vi "系统设置.vi"() -> ()   [LabVIEW 2016]
uses:
  <vilib>/Utility/miscctls.llb/LVPointTypeDef.ctl
  <vilib>/ptbypt/NI_PtbyPt.lvlib
  <vilib>/Utility/config.llb/NI_LVConfig.lvlib
  PLC/PLC.lvlib
panel:
  in  "CODCr":bool
  in  "总磷总氮":bool
  in  "氨氮":bool
  in  "CODmn":bool
  in  "多参数":bool
  in  "24H周期设置":bool[](xcontrol)
  in  "输入密码":dbl
  in  "布尔":bool
  in  "副屏设置":bool
  in  "开机启动":bool caption="氨氮禁用"
  in  "CODMn启用":bool caption="CODMn禁用"
  in  "质控单元启用":bool caption="质控单元禁用"
  in  "总磷总氮启用":bool caption="总磷总氮禁用"
  in  "流量计启用":bool caption="流量计禁用"
  in  "氨氮启用":bool caption="氨氮禁用"
  in  "多参数启用":bool caption="多参数禁用"
  in  "CODcr启用":bool caption="CODcr禁用"
  in  "运行模式":enum16{"维护模式", "常规模式", "应急模式", "质控模式"}(ring)
  # "自动运行启动参数"
  # "启动周期设置"
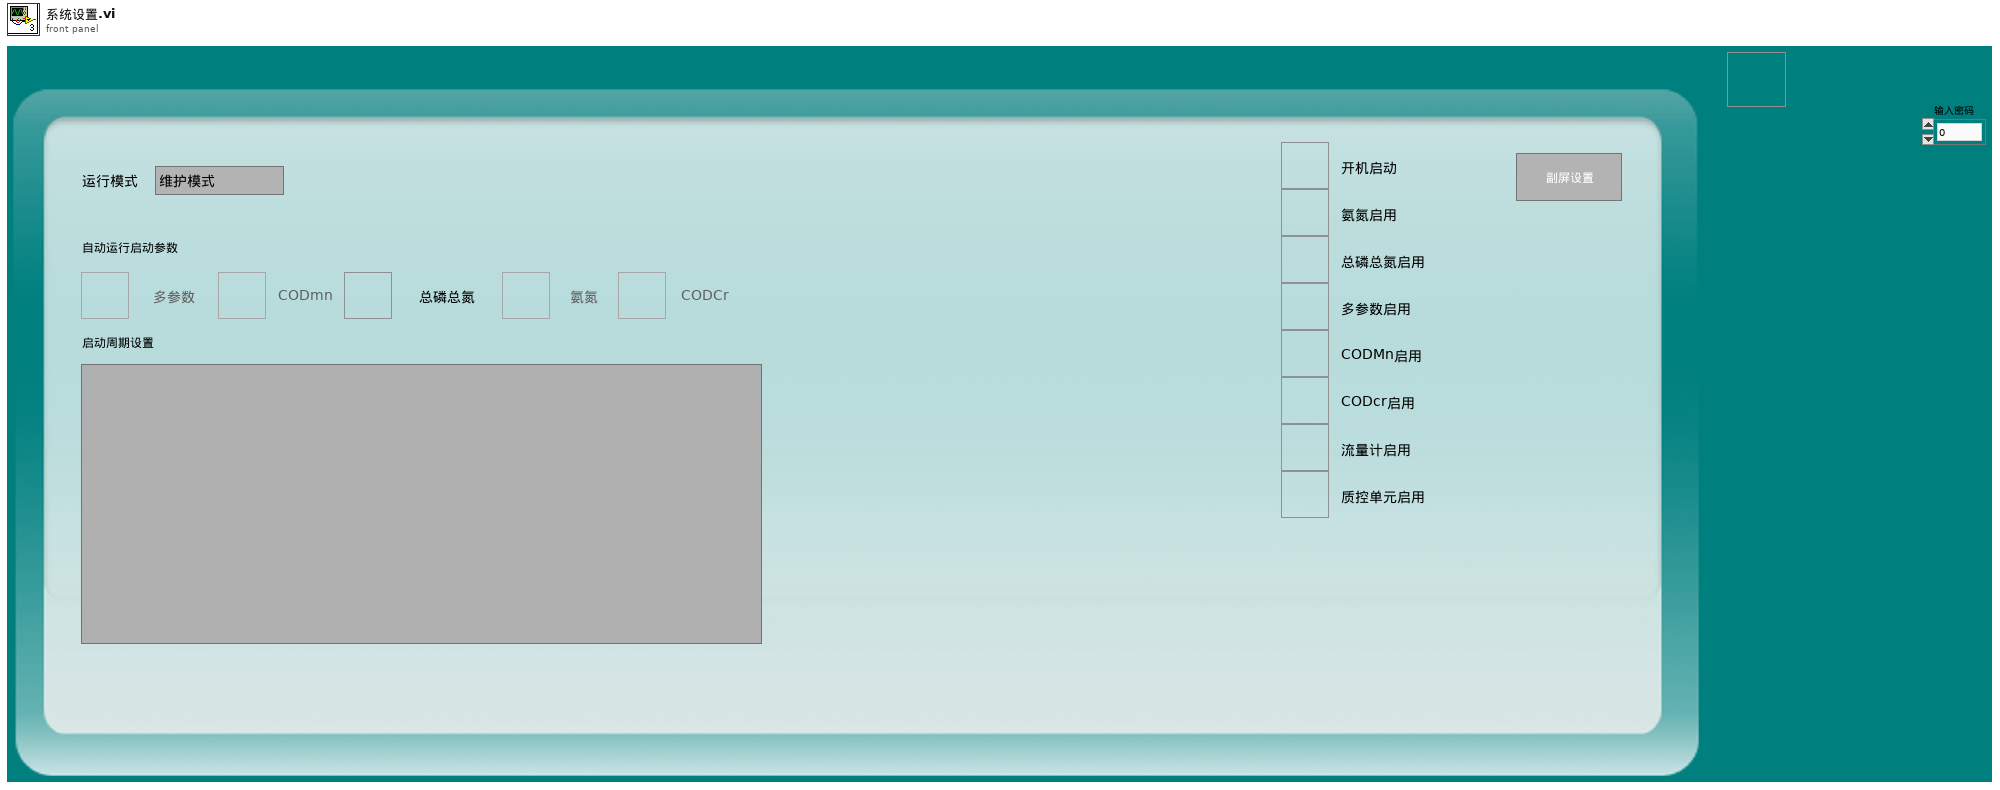
[diagram p1: front panel]
types:
  T1 = typedef "LVPointTypeDef.ctl" = cluster{"Horizontal":i16, "Vertical":i16}
  T2 = typedef "NI_LVConfig.lvlib/Config Data RefNum.ctl" = refnum<k1>
  T3 = enum8{"Enabled", "Disabled", "Disabled and Grayed Out"}
  T4 = cluster{"运行模式":enum16{"维护模式", "常规模式", "应急模式", "质控模式"}}
  T5 = cluster{"测量模式":enum16{"水样测量", "标样核查", "零点核查", "加标回收", "平行样", "校零", "校标"}}
  T6 = cluster{"CODCr":cluster{"启动测量模式":cluster{"测量模式":enum16{"水样测量", "标样核查", "零点核查", "加标回收", "平行样", "校零", "校标"}}, "确定按钮":bool}, "参数启用":cluster{"多参数":bool, "CODMn":bool, "总磷总氮":bool, "氨氮":bool, "CODcr":bool}}
  T7 = typedef "LVDateTimeRec.ctl" = cluster{"秒数的小数部分":dbl, "秒":i32, "分":i32, "时":i32, "日":i32, "月":i32, "年":i32, "天数（周）":i32, "天数（年）":i32, "DST":i32}
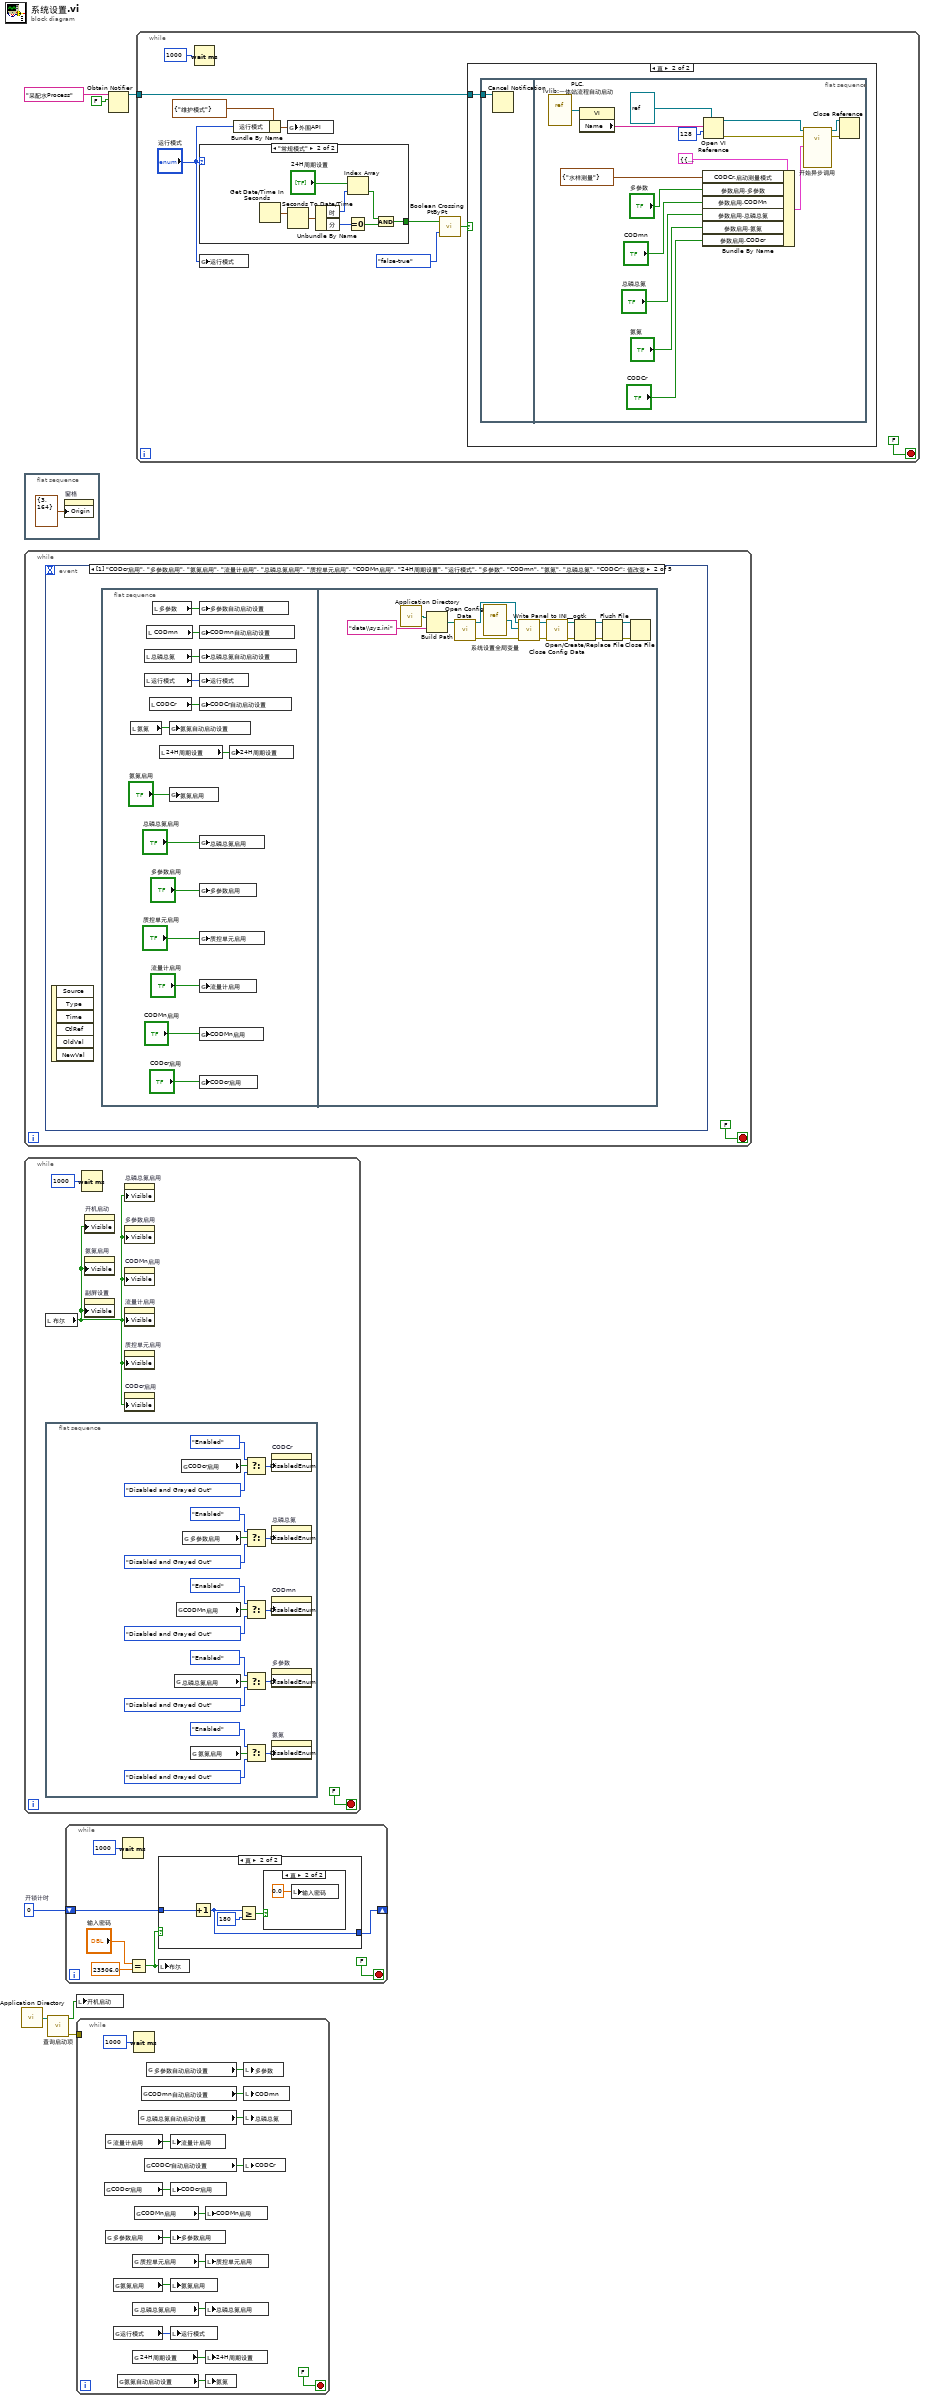
[diagram p0: block diagram]
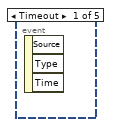
[diagram p6: hidden frame]
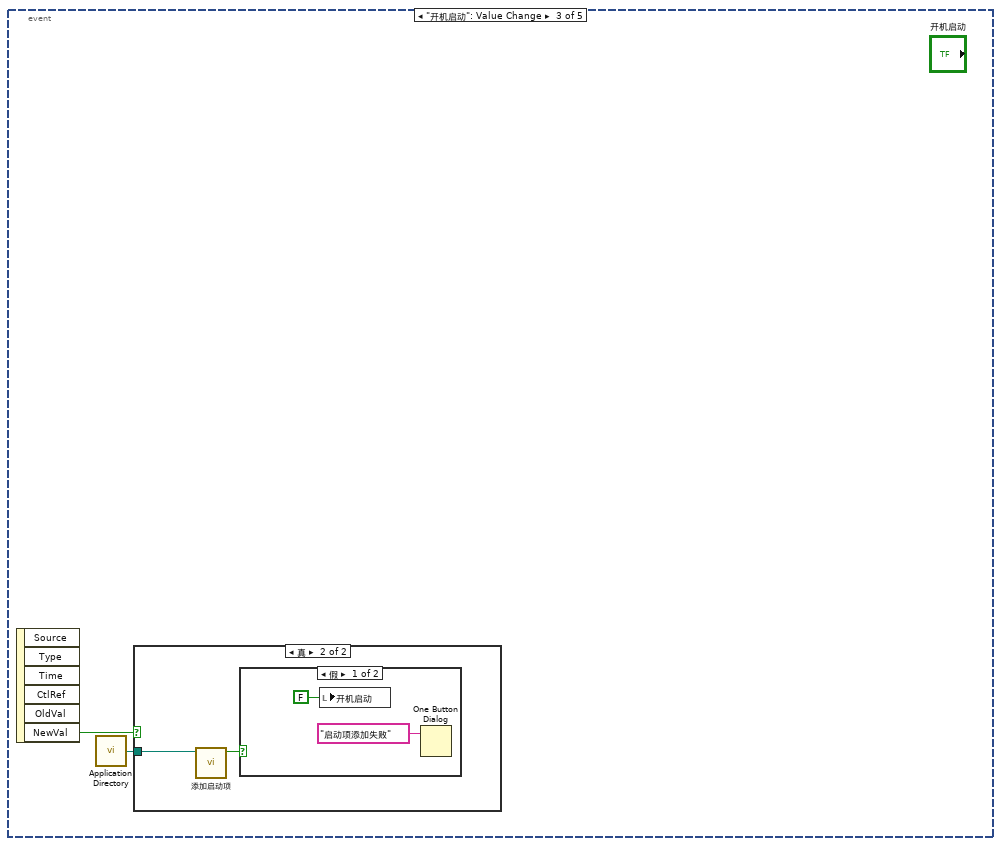
[diagram p7: hidden frame]
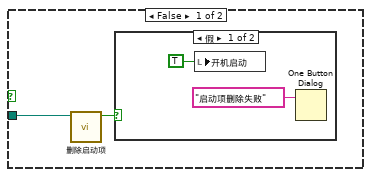
[diagram p8: hidden frame]
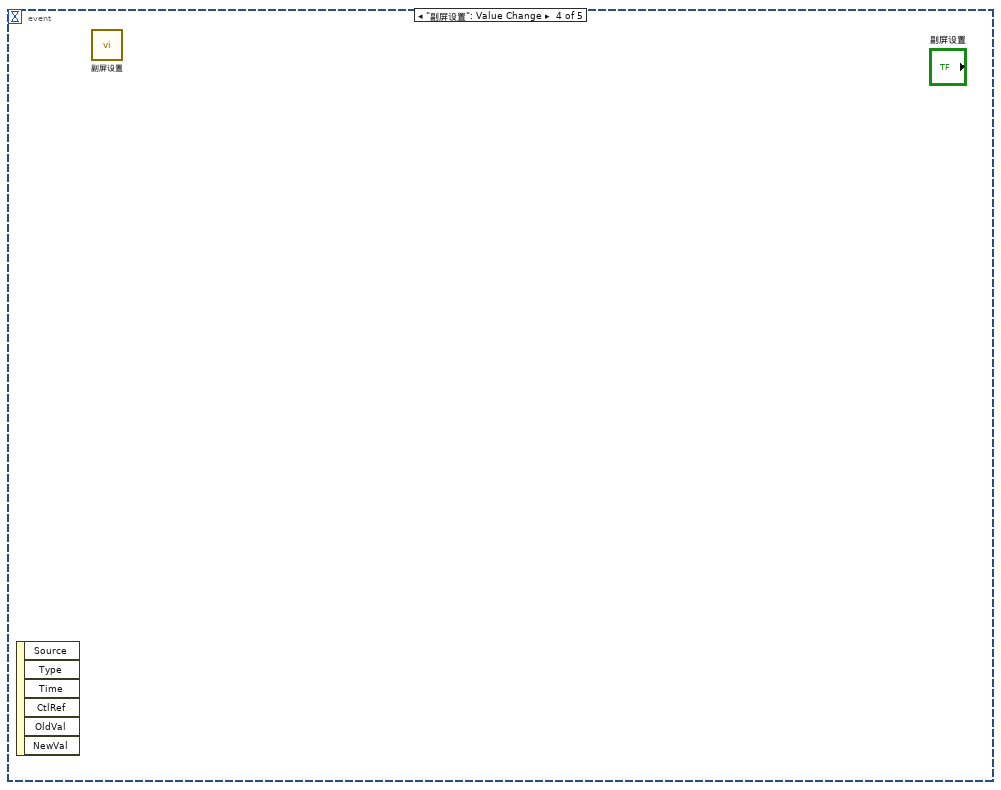
[diagram p11: hidden frame]
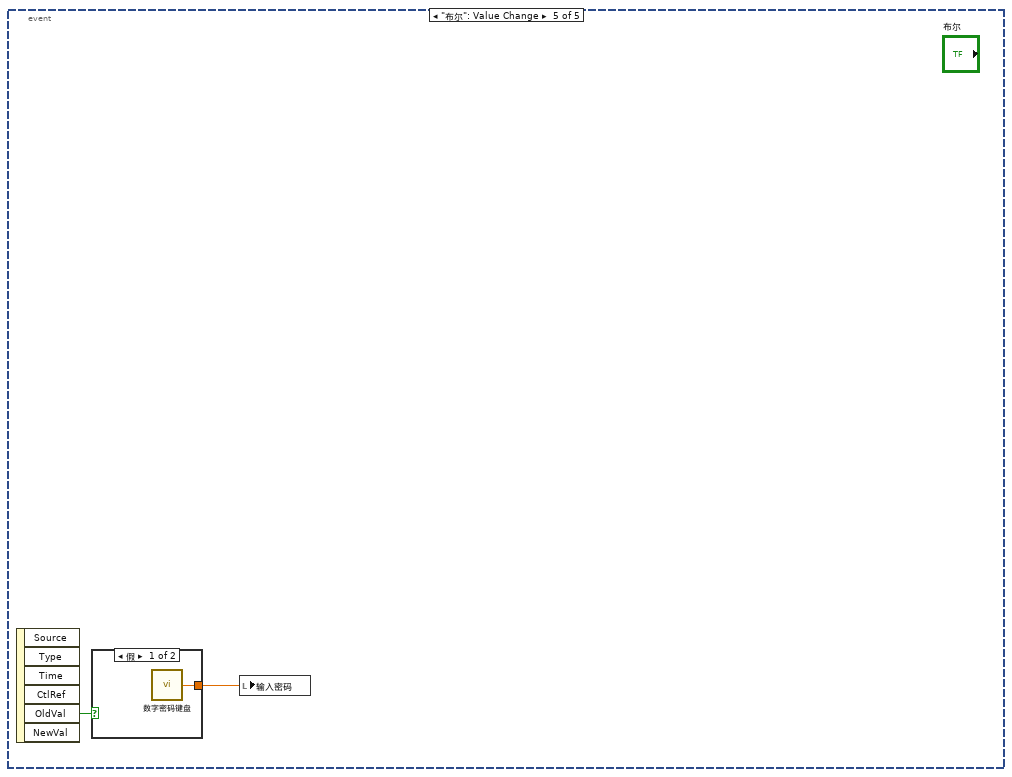
[diagram p12: hidden frame]
diagram:
  w1 = u32 0  # 开锁计时
  n1 = call <vilib>:"Application Directory.vi"() -> ("Application Directory"=w4:path)
  n2 = flat-sequence {
    frame #0 {
      n3 = property on="窗格" class="Pane"("Origin"=T1 {"Horizontal"=3, "Vertical"=164} ("原点")) -> ()  [unwired: 2 in, 2 out]
    }
  }
  n4 = while {
    stop <- FALSE stop-if-true
    n5 = event shown="[1] \"CODcr启用\", \"多参数启用\", \"氨氮启用\", \"流量计启用\", \"总磷总氮启用\", \"质控单元启用\", \"CODMn启用\", \"24H周期设置\", \"运行模式\", \"多参数\", \"CODmn\", \"氨氮\", \"总磷总氮\", \"CODCr\": 值改变" {
      selector: _ -> [_ _ _ _ _]
      dyn-events: _ -> [_ _ _ _ _]
      timeout: _ -> [_ _ _ _ _]
      event Timeout {
        n6 = event-data() -> ()  [unwired: 1 in, 3 out]
      }
      event "CODcr启用", "多参数启用", "氨氮启用", "流量计启用", "总磷总氮启用", "质控单元启用", "CODMn启用", "24H周期设置", "运行模式", "多参数", "CODmn", "氨氮", "总磷总氮", "CODCr": Value Change {
        n7 = event-data() -> ()  [unwired: 1 in, 6 out]
        n8 = flat-sequence {
          frame #0 {
            n9 = local read "氨氮"() -> (w14:bool)
            n10 = local read "总磷总氮"() -> (w12:bool)
            n11 = local read "运行模式"() -> (w15:enum16{"维护模式", "常规模式", "应急模式", "质控模式"})
            n12 = local read "CODmn"() -> (w11:bool)
            n13 = local read "CODCr"() -> (w13:bool)
            n14 = local read "多参数"() -> (w10:bool)
            n15 = local read "24H周期设置"() -> (w16:bool[])
            n16 = global write "系统设置全局变量.vi" "氨氮自动启动设置"(w14) -> ()
            n17 = global write "系统设置全局变量.vi" "氨氮启用"("氨氮启用") -> ()
            n18 = global write "系统设置全局变量.vi" "多参数自动启动设置"(w10) -> ()
            n19 = global write "系统设置全局变量.vi" "CODmn自动启动设置"(w11) -> ()
            n20 = global write "系统设置全局变量.vi" "总磷总氮自动启动设置"(w12) -> ()
            n21 = global write "系统设置全局变量.vi" "运行模式"(w15) -> ()
            n22 = global write "系统设置全局变量.vi" "CODCr自动启动设置"(w13) -> ()
            n23 = global write "系统设置全局变量.vi" "总磷总氮启用"("总磷总氮启用") -> ()
            n24 = global write "系统设置全局变量.vi" "多参数启用"("多参数启用") -> ()
            n25 = global write "系统设置全局变量.vi" "质控单元启用"("质控单元启用") -> ()
            n26 = global write "系统设置全局变量.vi" "流量计启用"("流量计启用") -> ()
            n27 = global write "系统设置全局变量.vi" "CODMn启用"("CODMn启用") -> ()
            n28 = global write "系统设置全局变量.vi" "CODcr启用"("CODcr启用") -> ()
            n29 = global write "系统设置全局变量.vi" "24H周期设置"(w16) -> ()
          }
          frame #1 {
            n30 = call <vilib>:"Application Directory.vi"() -> ("Application Directory"=w37:path)
            n31 = Build Path(base path=w37, name or relative path="data\\sys.ini" ("名称或相对路径")) -> (appended path=w35:path)
            n32 = call <vilib>:"Open Config Data.vi"("configuration file path"=w35) -> ("error out"=w31:errorcluster, "refnum"=w34:T2)  [unwired: 8 in, 1 out]
            n33 = vi-ref "系统设置全局变量.vi"() -> (w33:refnum<vi>)
            n34 = call <userlib>:"Write Panel to INI__ogtk.vi"("error in (no error)"=w31, "VI ref"=w33, "refnum"=w34) -> ("error out"=w30:errorcluster, "refnum out"=w32:T2)  [unwired: 7 in]
            n35 = call <vilib>:"Close Config Data.vi"("error in (no error)"=w30, "refnum"=w32) -> ("error out"=w25:errorcluster, "file path"=w24:path)  [unwired: 8 in]
            n36 = Open/Create/Replace File(file path (use dialog)=w24, error in=w25) -> (refnum out=w28:refnum<file>, error out=w29:errorcluster)  [unwired: 4 in, 1 out]
            n37 = Flush File(refnum=w28, error in=w29) -> (refnum out=w27:refnum<file>, error out=w26:errorcluster)
            n38 = Close File(refnum=w27, error in=w26) -> ()  [unwired: 2 out]
          }
        }
      }
      event "开机启动": Value Change {
        n39 = event-data() -> ("NewVal"=w39:bool)  [unwired: 1 in, 5 out]
        n40 = call <vilib>:"Application Directory.vi"() -> ("Application Directory"=w38:path)
        n41 = case shown="真" w39 {
          tunnel: w38 -> [w41 w45]
          frame False {
            n42 = call "删除启动项.vi"("启动文件路径"=w41) -> ("删除标记"=w40:bool)  [unwired: 9 in, 1 out]
            n43 = case shown="假" w40 {
              frame False {
                n44 = local write "开机启动"(TRUE ("开机启动")) -> ()
                n45 = One Button Dialog(message="启动项删除失败" ("消息")) -> ()  [unwired: 1 in, 1 out]
              }
              frame True {
              }
            }
          }
          frame True {
            n46 = call "添加启动项.vi"("启动文件路径"=w45) -> ("添加成功标记"=w44:bool)  [unwired: 9 in, 1 out]
            n47 = case shown="假" w44 {
              frame False {
                n48 = local write "开机启动"(FALSE ("开机启动")) -> ()
                n49 = One Button Dialog(message="启动项添加失败" ("消息")) -> ()  [unwired: 1 in, 1 out]
              }
              frame True {
              }
            }
          }
        }
      }
      event "副屏设置": Value Change {
        n50 = event-data() -> ()  [unwired: 1 in, 6 out]
        n51 = call "副屏设置.vi"() -> ()  [unwired: 12 in]
      }
      event "布尔": Value Change {
        n52 = event-data() -> ("OldVal"=w49:bool)  [unwired: 1 in, 5 out]
        n53 = case shown="假" w49 {
          tunnel: [w50 _] -> w48
          frame False {
            n54 = call "数字密码键盘.vi"() -> ("NewNumber"=w50:sgl)  [unwired: 1 in]
          }
          frame True {
          }
        }
        n55 = local write "输入密码"(w48) -> ()
      }
    }
  }
  n56 = while {
    stop <- FALSE stop-if-true
    n57 = local read "布尔"() -> (w51:bool)
    n58 = flat-sequence {
      frame #0 {
        n59 = global read "系统设置全局变量.vi" "总磷总氮启用"() -> (w58:bool)
        n60 = global read "系统设置全局变量.vi" "CODMn启用"() -> (w56:bool)
        n61 = global read "系统设置全局变量.vi" "CODcr启用"() -> (w57:bool)
        n62 = global read "系统设置全局变量.vi" "多参数启用"() -> (w55:bool)
        n63 = global read "系统设置全局变量.vi" "氨氮启用"() -> (w54:bool)
        n64 = Select(t=T3."Enabled" ("禁用"), s=w57, f=T3."Disabled and Grayed Out" ("禁用")) -> (s? t:f=w73:T3)
        n65 = Select(t=T3."Enabled" ("禁用"), s=w55, f=T3."Disabled and Grayed Out" ("禁用")) -> (s? t:f=w62:T3)
        n66 = Select(t=T3."Enabled" ("禁用"), s=w56, f=T3."Disabled and Grayed Out" ("禁用")) -> (s? t:f=w61:T3)
        n67 = Select(t=T3."Enabled" ("禁用"), s=w58, f=T3."Disabled and Grayed Out" ("禁用")) -> (s? t:f=w60:T3)
        n68 = Select(t=T3."Enabled" ("禁用"), s=w54, f=T3."Disabled and Grayed Out" ("禁用")) -> (s? t:f=w59:T3)
        n69 = property on="CODCr" class="Bool (严格)"("DisabledEnum"=w73) -> ()  [unwired: 2 in, 2 out]
        n70 = property on="总磷总氮" class="Bool (严格)"("DisabledEnum"=w62) -> ()  [unwired: 2 in, 2 out]
        n71 = property on="CODmn" class="Bool (严格)"("DisabledEnum"=w61) -> ()  [unwired: 2 in, 2 out]
        n72 = property on="多参数" class="Bool (严格)"("DisabledEnum"=w60) -> ()  [unwired: 2 in, 2 out]
        n73 = property on="氨氮" class="Bool (严格)"("DisabledEnum"=w59) -> ()  [unwired: 2 in, 2 out]
      }
    }
    n74 = Wait (ms)(milliseconds to wait=u32 1000 ("等待时间（毫秒）")) -> ()  [unwired: 1 out]
    n75 = property on="开机启动" class="Bool (严格)"("Visible"=w51) -> ()  [unwired: 2 in, 2 out]
    n76 = property on="氨氮启用" class="Bool (严格)"("Visible"=w51) -> ()  [unwired: 2 in, 2 out]
    n77 = property on="副屏设置" class="Bool"("Visible"=w51) -> ()  [unwired: 2 in, 2 out]
    n78 = property on="总磷总氮启用" class="Bool (严格)"("Visible"=w51) -> ()  [unwired: 2 in, 2 out]
    n79 = property on="多参数启用" class="Bool (严格)"("Visible"=w51) -> ()  [unwired: 2 in, 2 out]
    n80 = property on="CODMn启用" class="Bool (严格)"("Visible"=w51) -> ()  [unwired: 2 in, 2 out]
    n81 = property on="流量计启用" class="Bool (严格)"("Visible"=w51) -> ()  [unwired: 2 in, 2 out]
    n82 = property on="质控单元启用" class="Bool (严格)"("Visible"=w51) -> ()  [unwired: 2 in, 2 out]
    n83 = property on="CODcr启用" class="Bool (严格)"("Visible"=w51) -> ()  [unwired: 2 in, 2 out]
  }
  n84 = call "查询启动项.vi"("启动文件路径"=w4) -> ("error out"=w2:errorcluster, "包含启动项"=w3:bool)  [unwired: 9 in]
  n85 = while {
    shift-right: [w75] -> _
    shift-left: w1 -> [w76]
    stop <- FALSE stop-if-true
    n86 = Wait (ms)(milliseconds to wait=u32 1000 ("等待时间（毫秒）")) -> ()  [unwired: 1 out]
    n87 = Equal?(x="输入密码", y=23506.0) -> (x = y?=w74:bool)
    n88 = case shown="真" w74 {
      tunnel: w76 -> [_ w84]
      tunnel: [_ w83] -> w75
      frame False {
      }
      frame True {
        n89 = Increment(x=w84) -> (x+1=w83:u32)
        n90 = Greater Or Equal?(x=w83, y=u32 180) -> (x >= y?=w81:bool)
        n91 = case shown="真" w81 {
          frame False {
          }
          frame True {
            n92 = local write "输入密码"(0.0 ("输入密码")) -> ()
          }
        }
      }
    }
    n93 = local write "布尔"(w74) -> ()
  }
  n94 = local write "开机启动"(w3) -> ()
  n95 = while {
    tunnel: w2 -> [_]
    stop <- FALSE stop-if-true
    n96 = global read "系统设置全局变量.vi" "CODcr启用"() -> (w94:bool)
    n97 = global read "系统设置全局变量.vi" "流量计启用"() -> (w95:bool)
    n98 = global read "系统设置全局变量.vi" "多参数启用"() -> (w93:bool)
    n99 = global read "系统设置全局变量.vi" "氨氮启用"() -> (w99:bool)
    n100 = global read "系统设置全局变量.vi" "运行模式"() -> (w91:enum16{"维护模式", "常规模式", "应急模式", "质控模式"})
    n101 = global read "系统设置全局变量.vi" "氨氮自动启动设置"() -> (w90:bool)
    n102 = global read "系统设置全局变量.vi" "质控单元启用"() -> (w97:bool)
    n103 = global read "系统设置全局变量.vi" "总磷总氮启用"() -> (w96:bool)
    n104 = global read "系统设置全局变量.vi" "24H周期设置"() -> (w92:bool[])
    n105 = Wait (ms)(milliseconds to wait=u32 1000 ("等待时间（毫秒）")) -> ()  [unwired: 1 out]
    n106 = global read "系统设置全局变量.vi" "CODMn启用"() -> (w98:bool)
    n107 = global read "系统设置全局变量.vi" "总磷总氮自动启动设置"() -> (w88:bool)
    n108 = global read "系统设置全局变量.vi" "CODmn自动启动设置"() -> (w87:bool)
    n109 = global read "系统设置全局变量.vi" "CODCr自动启动设置"() -> (w89:bool)
    n110 = global read "系统设置全局变量.vi" "多参数自动启动设置"() -> (w86:bool)
    n111 = local write "流量计启用"(w95) -> ()
    n112 = local write "CODcr启用"(w94) -> ()
    n113 = local write "多参数启用"(w93) -> ()
    n114 = local write "氨氮启用"(w99) -> ()
    n115 = local write "运行模式"(w91) -> ()
    n116 = local write "CODMn启用"(w98) -> ()
    n117 = local write "质控单元启用"(w97) -> ()
    n118 = local write "总磷总氮启用"(w96) -> ()
    n119 = local write "24H周期设置"(w92) -> ()
    n120 = local write "氨氮"(w90) -> ()
    n121 = local write "多参数"(w86) -> ()
    n122 = local write "CODmn"(w87) -> ()
    n123 = local write "总磷总氮"(w88) -> ()
    n124 = local write "CODCr"(w89) -> ()
  }
  n125 = Obtain Notifier(name (unnamed)="采配水Process" ("名称（未命名）"), notification data type=FALSE) -> (notifier out=w5:refnum<notifier>)  [unwired: 2 in, 2 out]
  n126 = while {
    tunnel: w5 -> [w108]
    stop <- FALSE stop-if-true
    n127 = Wait (ms)(milliseconds to wait=u32 1000 ("等待时间（毫秒）")) -> ()  [unwired: 1 out]
    n128 = case shown="\"常规模式\"" "运行模式" {
      tunnel: [_ w132] -> w107
      frame "维护模式", Default {
      }
      frame "常规模式" {
        n129 = Get Date/Time In Seconds() -> (seconds since 1Jan1904=w136:timestamp)
        n130 = Seconds To Date/Time(time stamp (now)=w136) -> (date time rec=w135:T7)  [unwired: 1 in]
        n131 = Unbundle By Name(w135) -> ("时"=w130:i32, "分"=w134:i32)
        n132 = Equal To 0?(x=w134) -> (x = 0?=w133:bool)
        n133 = Index Array(array="24H周期设置", index=w130) -> (element=w129:bool)
        n134 = And(x=w129, y=w133) -> (x .and. y?=w132:bool)
      }
    }
    n135 = global write "系统变量.vi" "运行模式"("运行模式") -> ()
    n136 = Bundle By Name(cluster=T4 {"运行模式"=enum."维护模式"} ("外围API"), "运行模式"="运行模式") -> (w103:T4)
    n137 = global write "VAR总磷氨氮全局变量.vi" "外围API"(w103) -> ()
    n138 = call <vilib>:"Boolean Crossing PtByPt.vi"("direction"=enum16{"either", "false-true", "true-false"}."false-true", "input"=w107) -> ("crossing"=w105:bool)  [unwired: 1 in]
    n139 = case shown="真" w105 {
      tunnel: w108 -> [_ w111]
      frame False {
      }
      frame True {
        n140 = flat-sequence {
          tunnel: w111 -> [w112]
          frame #0 {
            n141 = Cancel Notification(0:w112) -> ()  [unwired: 1 in, 3 out]
          }
          frame #1 {
            n142 = vi-ref "PLC.lvlib:一体站流程自动启动.vi"() -> (w128:refnum<vi>)
            n143 = property class="VI"(reference=w128) -> ("Name"=w127:string)  [unwired: 1 in, 2 out]
            n144 = Bundle By Name(cluster=T6 {"CODCr"={"启动测量模式"={"测量模式"=enum."水样测量"}, "确定按钮"=TRUE}, "参数启用"={"多参数"=FALSE, "CODMn"=FALSE, "总磷总氮"=FALSE, "氨氮"=FALSE, "CODcr"=FALSE}} ("参数"), "CODCr.启动测量模式"=T5 {"测量模式"=enum."水样测量"}, "参数启用.多参数"="多参数", "参数启用.CODMn"="CODmn", "参数启用.总磷总氮"="总磷总氮", "参数启用.氨氮"="氨氮", "参数启用.CODcr"="CODCr") -> (w118:T6)
            n145 = Open VI Reference(type specifier VI Refnum (for type only)=refnum<vi> refnum, vi path=w127, options=128 ("选项")) -> (vi reference=w125:refnum<vi>, error out=w122:errorcluster)  [unwired: 3 in]
            n146 = call-by-ref "开始异步调用"(reference=w125, error in=w122, "参数"=w118) -> (reference out=w123:refnum<vi>, error out=w121:errorcluster)  [unwired: 11 in]
            n147 = Close Reference(reference=w123, error in (no error)=w121) -> ()  [unwired: 1 out]
          }
        }
      }
    }
  }
